vi "Eth Status Write Stop_com.vi"(7 "Status Reference":T1, 8 "error in (no error)":errorcluster, 10 "Stop":bool) -> (0 "error out":errorcluster)   [LabVIEW 2021, in "Eth Status.lvlib"]
uses:
  Eth Status.lvlib
  Ctl/Status.ctl
  MB_TCP2/MB_TCP_State.ctl
  MB_TCP2/MB_TCP.lvclass
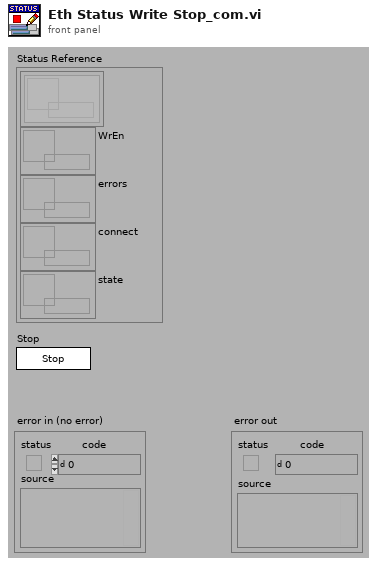
[diagram p1: front panel]
types:
  T1 = typedef "Eth Status.lvlib/Status.ctl" = cluster{"Set_states":refnum<queue>[], "WrEn":refnum<data-value>, "errors":refnum<data-value>, "connect":refnum<data-value>, "state":refnum<data-value>}
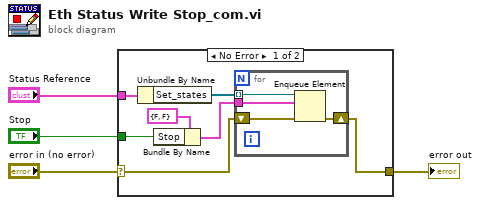
[diagram p0: block diagram]
diagram:
  n1 = case shown="No Error" "error in (no error)" {
    selector: "error in (no error)" -> [w5 w16]
    tunnel: "Status Reference" -> [w11 _]
    tunnel: "Stop" -> [w8 _]
    tunnel: [w6 w16] -> w2
    frame No Error {
      n2 = Unbundle By Name(w11) -> ("Set_states"=w9:refnum<queue>[])
      n3 = Bundle By Name(cluster=cluster{"Start":bool, "Stop":bool} {"Start"=FALSE, "Stop"=FALSE} ("element"), "Stop"=w8) -> (w10:cluster{"Start":bool, "Stop":bool})
      n4 = for {
        tunnel: w9 -> [w15] mode=indexing
        tunnel: w10 -> [w12]
        shift-right: [w13] -> w6
        shift-left: w5 -> [w14]
        n5 = Enqueue Element(queue=w15, element=w12, error in (no error)=w14) -> (error out=w13:errorcluster)  [unwired: 1 in, 2 out]
      }
    }
    frame Error {
    }
  }
  "error out" <- w2
